vi "Set_Iterations.vi"(1 "Iterations":u32, 2 "Index":i32, 3 "Input Sequence":cluster{string, string[], dbl[], dbl}[](array[cluster])) -> (0 "Output Sequence":cluster{string, string[], dbl[], dbl}[](array[cluster]))   [LabVIEW 2011]
doc: "This VI sets the desired number of iterations of an event in the sequence given by the \"Index\" parameter."
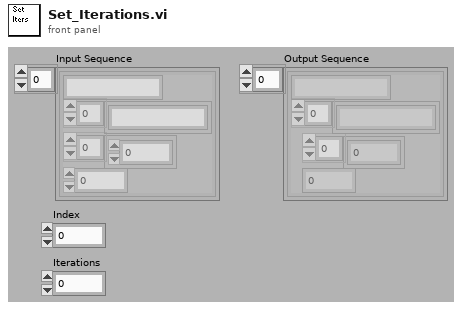
[diagram p1: front panel]
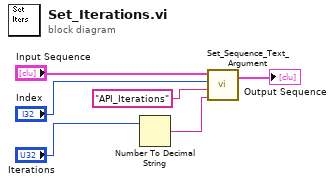
[diagram p0: block diagram]
diagram:
  n1 = Number To Decimal String(number="Iterations") -> (decimal integer string=w1:string)  [unwired: 1 in]
  n2 = call "Set_Sequence_Text_Argument.vi"("Text"=w1, "Argument"="API_Iterations", "Index"="Index", "Input Sequence"="Input Sequence") -> ("Output Sequence"=→"Output Sequence":cluster{string, string[], dbl[], dbl}[])  [unwired: 1 out]
